vi "AutoRotate.vi"(6 "BreakScaler":dbl=1.0 min=0.0 step=0.1, 8 "AccelRate":dbl, 9 "Actual":dbl, 10 "Desired":dbl) -> (2 "Right":dbl, 3 "Left":dbl)   [LabVIEW 2013]
doc: "The quickest and most efficient algorithm for automatically rotating the robot to a given orientation. Remember, winners us this VI."
uses:
  Robot Global Data.vi
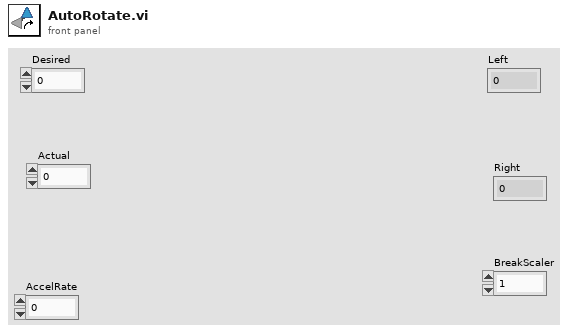
[diagram p1: front panel]
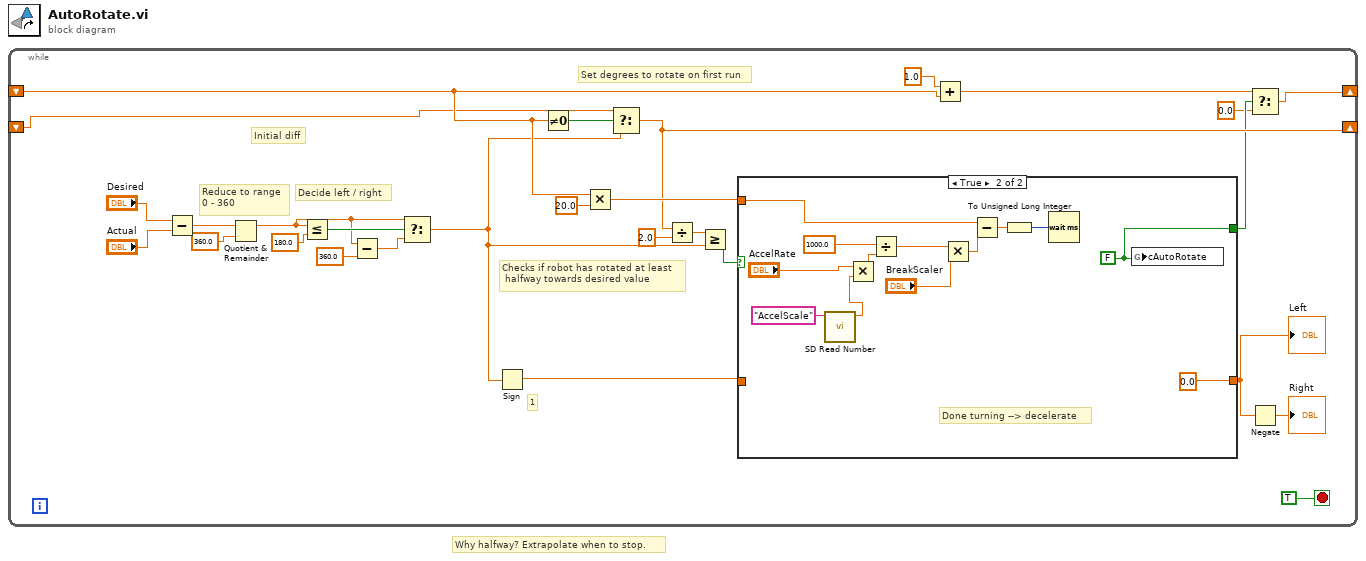
[diagram p0: block diagram]
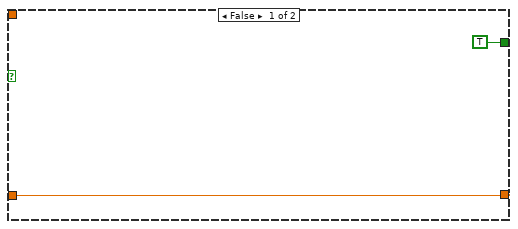
[diagram p2: hidden frame]
diagram:
  # "Why halfway? Extrapolate when to stop."
  n1 = while {
    shift-right: [w5] -> _
    shift-left: _ -> [w7]
    shift-right: [w2] -> _
    shift-left: _ -> [w11]
    stop <- TRUE stop-if-true
    # "Reduce to range\n0 - 360"
    # "Decide left / right"
    # "1"
    # "Initial diff"
    # "Set degrees to rotate on first run"
    # "Checks if robot has rotated at least\n halfway towards desired value"
    n2 = Subtract(x="Desired", y="Actual") -> (x-y=w21:dbl)
    n3 = Quotient & Remainder(x=w21, y=360.0) -> (x-y*floor(x/y)=w16:dbl)  [unwired: 1 out]
    n4 = Less Or Equal?(x=w16, y=180.0) -> (x <= y?=w18:bool)
    n5 = Subtract(x=w16, y=360.0) -> (x-y=w17:dbl)
    n6 = Select(t=w16, s=w18, f=w17) -> (s? t:f=w6:dbl)
    n7 = Sign(1:w6) -> (0:w15:dbl)
    n8 = Not Equal To 0?(x=w11) -> (x != 0?=w8:bool)
    n9 = Multiply(x=w11, y=20.0) -> (x*y=w25:dbl)
    n10 = Select(t=w7, s=w8, f=w6) -> (s? t:f=w5:dbl)
    n11 = Divide(x=w5, y=2.0) -> (x/y=w14:dbl)
    n12 = Greater Or Equal?(x=w14, y=w6) -> (x >= y?=w23:bool)
    n13 = case shown="True" w23 {
      tunnel: [w30 0.0] -> w9
      tunnel: w25 -> [_ w42]
      tunnel: w15 -> [w30 _]
      tunnel: [TRUE w34] -> w4
      frame False {
      }
      frame True {
        w34 = FALSE
        # "Done turning --> decelerate"
        n14 = call <vilib>:"SD Read Number.vi"("Name"="AccelScale") -> ("Numeric"=w37:dbl)  [unwired: 8 in, 2 out]
        n15 = Multiply(x="AccelRate", y=w37) -> (x*y=w38:dbl)
        n16 = Divide(x=1000.0, y=w38) -> (x/y=w33:dbl)
        n17 = Multiply(x=w33, y="BreakScaler") -> (x*y=w31:dbl)
        n18 = Subtract(x=w42, y=w31) -> (x-y=w41:dbl)
        n19 = To Unsigned Long Integer(number=w41) -> (unsigned 32bit integer=w35:u32)
        n20 = Wait (ms)(milliseconds to wait=w35) -> ()  [unwired: 1 out]
        n21 = global write "Robot Global Data.vi" "cAutoRotate"(w34) -> ()
      }
    }
    "Left" <- w9
    n22 = Add(x=1.0, y=w11) -> (x+y=w3:dbl)
    n23 = Select(t=w3, s=w4, f=0.0) -> (s? t:f=w2:dbl)
    n24 = Negate(x=w9) -> (-x=→"Right":dbl)
  }
